vi "Connection Handler.vi"(6 "connection reference":refnum<data-value>, 8 "UUID":string, 9 "Data Model":refnum<class "Device Data Model.lvclass">, 11 "TCP Server":refnum<class "TCP Server.lvclass">) -> ()   [LabVIEW 2021, in "WebSockets.lvlib" / "TCP Server.lvclass"]
doc: "Handles new connections by waiting on TCP requests. When data is received, it will execute the modbus data unit and write the return data back onto the bus. It handles one request at a time."
uses:
  TCP Server.lvclass
  D:/my_projects/projects/21/WebSockets/Source/WebSockets/WebSocket/WebSocket.lvclass
  Connection.ctl
  Modbus_v121c/Data Model/Device Data Model.lvclass
  TCP Server.lvclass/TCP Server.ctl
  WebSocket/WebSocket.lvclass/WebSocket.ctl
  Data Model/WebSocket Data Model.lvclass
  Data Model/WebSocket Data Model.lvclass/WebSocket Data Model.ctl
  WebSocket/Opcodes.ctl
  Handler State.ctl
  WebSocket/Low-Level Write.vi
  WebSocket/Low-Level Read.vi
  Timing/Calculate Timeout.vi
  WebSocket/Pong.vi
  Timing/Tick Count with Error Wires.vi
  WebSocket/DataLengthBytes.vi
  WebSocket/EncodeMaskedBytes.vi
  WebSocket/Socket Write.vi
  WebSocket/Socket Read.vi
  <vilib>/Utility/error.llb/Error Cluster From Error Code.vi
  WebSocket/DecodeMaskedBytes.vi
  WebSocket/WebSocket.lvclass
  Sockets/Socket/Socket.lvclass
panel:
  out "error out":errorcluster
  out "Data":u8[](array[numeric])
  in  "stop":bool
  # "ToDo: Delete indicator"
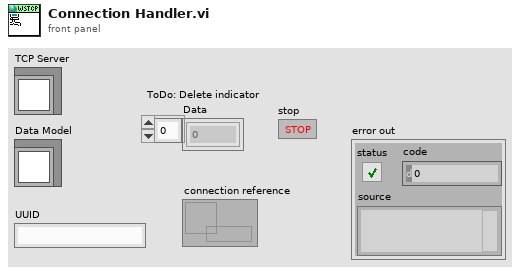
[diagram p1: front panel]
types:
  T1 = typedef "WebSockets.lvlib/WebSocket.lvclass/Opcodes.ctl" = u8
  T2 = typedef "WebSockets.lvlib/TCP Server.lvclass/Handler State.ctl" = enum16{"Wait on Connection", "Execute function", "Close Connection", "Quit"}
  T3 = typedef "WebSockets.lvlib/TCP Server.lvclass/Connection.ctl" = cluster{"Connected?":bool, "IP address":string, "connection error":errorcluster}
  T4 = typedef "WebSockets.lvlib/TCP Server.lvclass/Connection Counter.ctl" = cluster{"Currently Connected":u32, "Connection Records":refnum<data-value>[]}
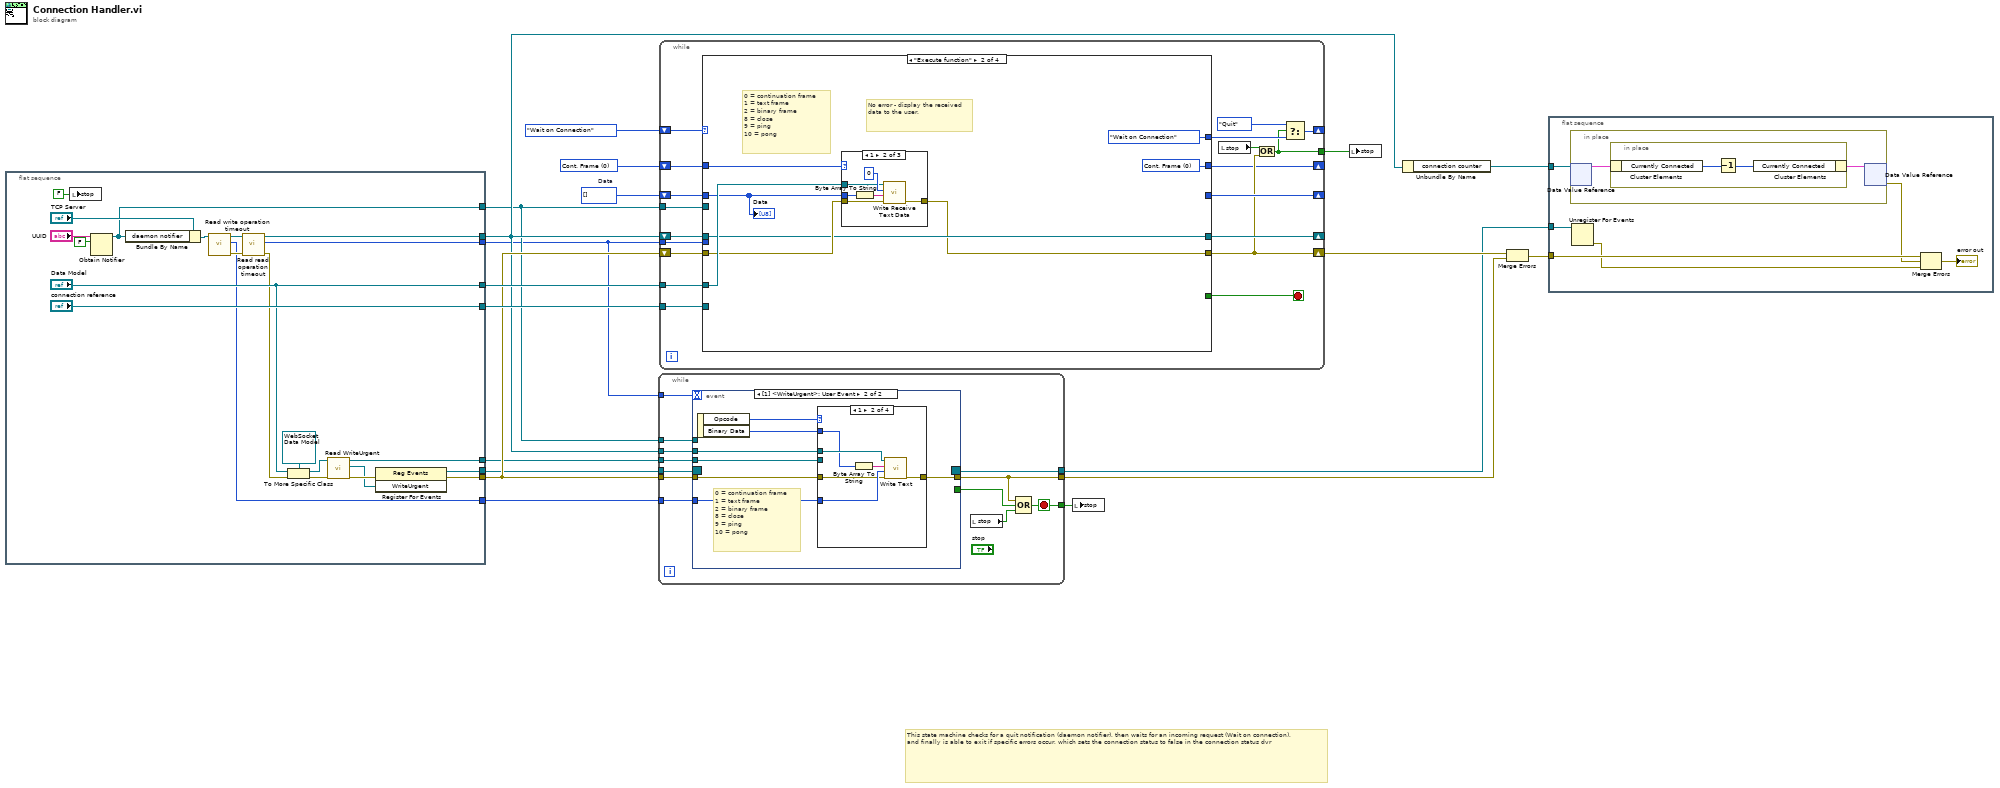
[diagram p0: block diagram]
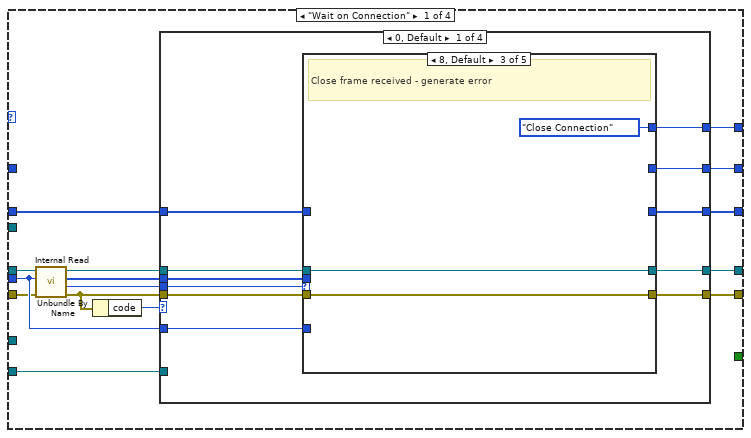
[diagram p2: hidden frame]
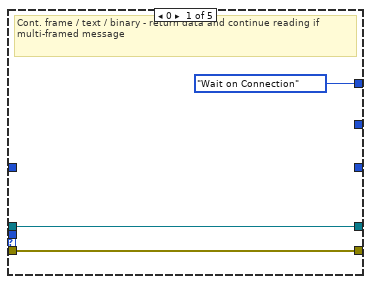
[diagram p3: hidden frame]
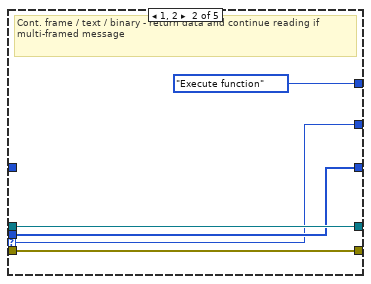
[diagram p4: hidden frame]
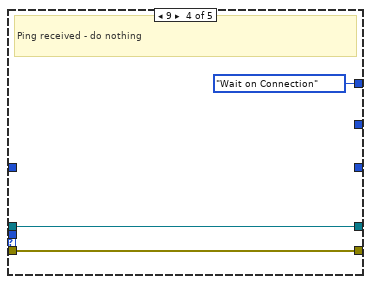
[diagram p5: hidden frame]
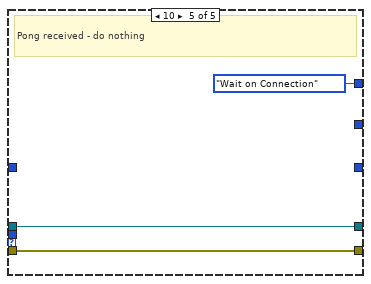
[diagram p6: hidden frame]
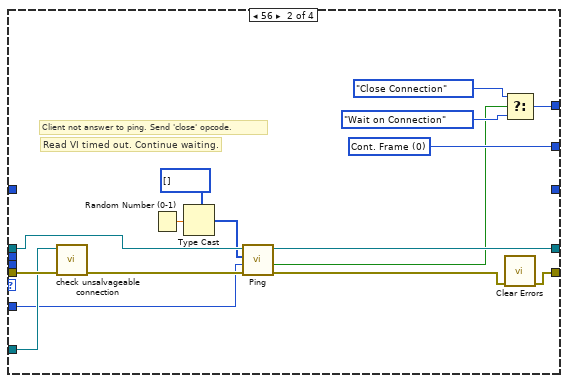
[diagram p7: hidden frame]
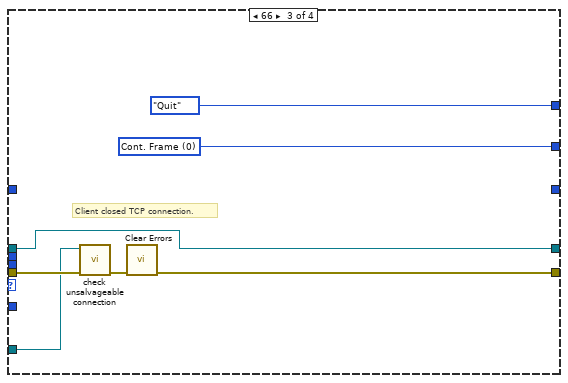
[diagram p8: hidden frame]
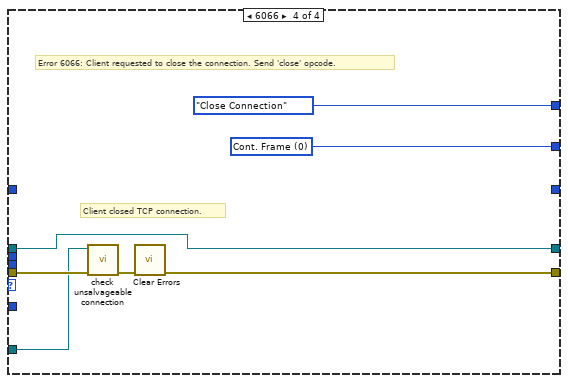
[diagram p9: hidden frame]
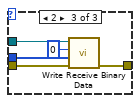
[diagram p11: hidden frame]
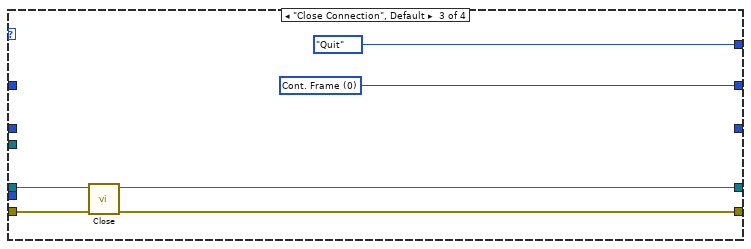
[diagram p12: hidden frame]
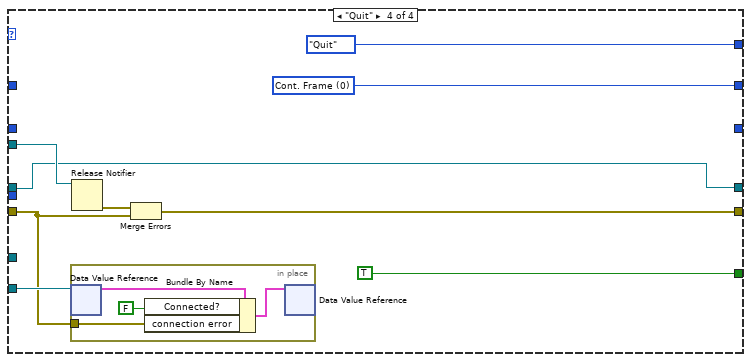
[diagram p13: hidden frame]
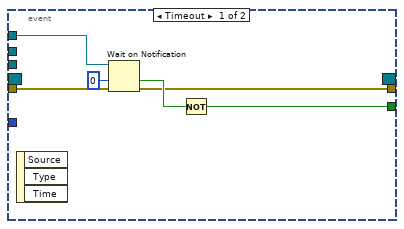
[diagram p14: hidden frame]
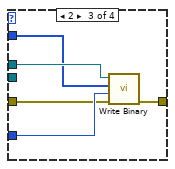
[diagram p16: hidden frame]
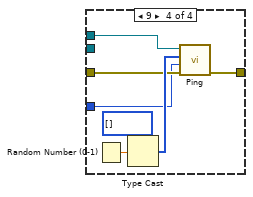
[diagram p17: hidden frame]
diagram:
  w5 = T1 0 items=["Cont. Frame"=0, "Text"=1, "Binary"=2, "Close Frame"=8, "Ping"=9, "Pong"=10] ("Opcode")
  w18 = u8[] []  # Data
  # "This state machine checks for a quit notification (daemon notifier), then waits for an incoming request (Wait on connection), and finally is able to exit if specific errors occur, which sets the connection status to false in the connection status dvr"
  n1 = flat-sequence {
    tunnel: ["connection reference"] -> w16
    tunnel: [w21] -> w12
    tunnel: [w36] -> w3
    tunnel: [w29] -> w11
    tunnel: [w35] -> w4
    tunnel: ["Data Model"] -> w13
    tunnel: [w20] -> w6
    tunnel: [w26] -> w9
    tunnel: [w24] -> w10
    frame #0 {
      n2 = local write "stop"(FALSE ("stop")) -> ()
      n3 = Obtain Notifier(name (unnamed)="UUID", notification data type=FALSE) -> (notifier out=w35:refnum<notifier>)  [unwired: 2 in, 2 out]
      n4 = Bundle By Name(cluster="TCP Server", "daemon notifier"=w35) -> (w30:refnum<class "TCP Server.lvclass">)
      n5 = call "Read write operation timeout.vi"("Socket in"=w30) -> ("error out"=w27:errorcluster, "write operation timeout"=w26:i32, "Socket out"=w28:refnum<class "TCP Server.lvclass">)  [unwired: 8 in]
      n6 = call "Read read operation timeout.vi"("error in (no error)"=w27, "Socket in"=w28) -> ("error out"=w25:errorcluster, "read operation timeout"=w36:i32, "Socket out"=w29:refnum<class "TCP Server.lvclass">)  [unwired: 7 in]
      n7 = To More Specific Class(target class=refnum<class "WebSocket Data Model.lvclass"> refnum ("WebSockets.lvlib:Device Data Model"), reference="Data Model", error in=w25) -> (specific class reference=w32:refnum<class "WebSocket Data Model.lvclass">, error out=w31:errorcluster)
      n8 = call "Read WriteUrgent.vi"("error in (no error)"=w31, "WebSocket Data Model in"=w32) -> ("error out"=w23:errorcluster, "WriteUrgent"=w22:refnum<user-event>, "WebSocket Data Model out"=w24:refnum<class "WebSocket Data Model.lvclass">)  [unwired: 7 in]
      n9 = register-events(error in=w23, w22) -> (reference out=w20:refnum<event-registration>, error out=w21:errorcluster)  [unwired: 1 in]
    }
  }
  n10 = while {
    tunnel: [w52] -> w8
    tunnel: [w43] -> w7
    tunnel: w6 -> [w47]
    tunnel: w12 -> [w51]
    tunnel: w11 -> [w50]
    tunnel: w10 -> [w49]
    tunnel: w9 -> [w48]
    tunnel: w4 -> [w46]
    tunnel: w3 -> [w45]
    tunnel: [w42] -> w2
    stop <- w52 stop-if-true
    n11 = event shown="[1] <WriteUrgent>: User Event" {
      selector: w47 -> [_ _]
      dyn-events: [_ _] -> w42
      timeout: w45 -> [_ _]
      tunnel: w51 -> [w56 w62]
      tunnel: w50 -> [_ w66]
      tunnel: w49 -> [_ w65]
      tunnel: [w55 w64] -> w43
      tunnel: w48 -> [_ w63]
      tunnel: w46 -> [w59 _]
      tunnel: [w57 _] -> w44
      event Timeout {
        n12 = event-data() -> ()  [unwired: 1 in, 3 out]
        n13 = Wait on Notification(notifier=w59, timeout in ms (-1)=0, error in (no error)=w56) -> (timed out?=w58:bool, error out=w55:errorcluster)  [unwired: 1 in, 2 out]
        n14 = Not(x=w58) -> (.not. x?=w57:bool)
      }
      event User Event {
        # "0 = continuation frame\n1 = text frame\n2 = binary frame\n8 = close\n9 = ping\n10 = pong"
        n15 = event-data() -> ("Opcode"=w61:T1, "Binary Data"=w60:u8[])  [unwired: 1 in]
        n16 = case shown="1" w61 {
          tunnel: w66 -> [_ w73 w78 w83]
          tunnel: w62 -> [w67 w69 w74 w81]
          tunnel: w65 -> [_ _ _ _]
          tunnel: w63 -> [_ w72 w76 w79]
          tunnel: [w67 w71 w77 w80] -> w64
          tunnel: w60 -> [_ w70 w75 _]
          frame 0, Default {
          }
          frame 1 {
            n17 = Byte Array To String(unsigned byte array=w70) -> (string=w68:string)
            n18 = call-dynamic "Write Text.vi"("error in (no error)"=w69, "timeout ms (5000)"=w72, "String Data"=w68, "WebSocket in"=w73) -> ("error out"=w71:errorcluster)  [unwired: 6 in, 1 out]
          }
          frame 2 {
            n19 = call-dynamic "Write Binary.vi"("error in (no error)"=w74, "timeout ms (5000)"=w76, "Binary Data"=w75, "WebSocket in"=w78) -> ("error out"=w77:errorcluster)  [unwired: 6 in, 1 out]
          }
          frame 9 {
            n20 = Random Number (0-1)() -> (number: 0 to 1=w84:dbl)
            n21 = Type Cast(type=u8[] [] ("values"), x=w84) -> (*(type *) &x=w82:u8[])
            n22 = call "Ping.vi"("error in (no error)"=w81, "timeout ms (5000)"=w79, "Payload"=w82, "WebSocket in"=w83) -> ("error out"=w80:errorcluster)  [unwired: 5 in, 2 out]
          }
        }
      }
    }
    n23 = local read "stop"() -> (w53:bool)
    n24 = Compound Arithmetic op=OR(w43, w44, w53) -> (w52:bool)
  }
  n25 = while {
    tunnel: w3 -> [w102]
    shift-right: [w103] -> _
    shift-left: w11 -> [w104]
    shift-right: [w100] -> _
    shift-left: w18 -> [w101]
    shift-right: [w91] -> _
    shift-left: Handler_State."Wait on Connection" ("Listener State") -> [w98]
    tunnel: w16 -> [w99]
    tunnel: w4 -> [w96]
    tunnel: [w89] -> w15
    shift-right: [w90] -> w14
    shift-left: w12 -> [w97]
    tunnel: w13 -> [w88]
    shift-right: [w87] -> _
    shift-left: w5 -> [w86]
    stop <- w95 stop-if-true
    n26 = case shown="\"Execute function\"" w98 {
      tunnel: w104 -> [w112 w181 w202 w207]
      tunnel: [w119 w180 w199 w211] -> w90
      tunnel: [w118 w181 w200 w207] -> w103
      tunnel: [_ _ _ TRUE ("Finished?")] -> w95
      tunnel: w102 -> [w109 _ _ _]
      tunnel: w101 -> [w117 w183 _ _]
      tunnel: [w116 _ _ _] -> w100
      tunnel: w99 -> [w114 _ _ w209]
      tunnel: [w113 Handler_State."Wait on Connection" ("Listener State") Handler_State."Quit" ("Listener State") Handler_State."Quit" ("Listener State")] -> w92
      tunnel: w97 -> [w108 w182 w203 w205]
      tunnel: w96 -> [_ _ _ w210]
      tunnel: w88 -> [_ w184 _ _]
      tunnel: [w105 w179 w198 w204] -> w87
      tunnel: w86 -> [_ w178 _ _]
      frame "Wait on Connection" {
        n27 = call "Internal Read.vi"("error in (no error)"=w108, "timeout ms"=w109, "WebSocket in"=w112) -> ("error out"=w107:errorcluster, "Opcode"=w106:T1, "Data"=w110:u8[], "WebSocket out"=w111:refnum<class "TCP Server.lvclass">)  [unwired: 5 in]
        n28 = Unbundle By Name(w107) -> ("code"=w115:i32)
        n29 = case shown="0, Default" w115 {
          tunnel: w107 -> [w130 w163 w169 w176]
          tunnel: [w129 w161 w167 w174] -> w119
          tunnel: w111 -> [w128 w160 w166 w173]
          tunnel: w110 -> [w127 _ _ _]
          tunnel: [w126 w149 w166 w173] -> w118
          tunnel: w106 -> [w125 _ _ _]
          tunnel: w109 -> [w124 w158 _ _]
          tunnel: w117 -> [w123 _ _ _]
          tunnel: [w122 _ _ _] -> w116
          tunnel: w114 -> [_ w162 w168 w175]
          tunnel: [w121 w155 Handler_State."Quit" ("Listener State") Handler_State."Close Connection" ("Listener State")] -> w113
          tunnel: [w120 w154 w164 w171] -> w105
          frame 0, Default {
            n30 = case shown="8, Default" w125 {
              selector: w125 -> [_ w134 _ _ _]
              tunnel: w130 -> [w132 w137 w141 w142 w146]
              tunnel: [w132 w137 w141 w142 w146] -> w129
              tunnel: w128 -> [w133 w138 w140 w143 w147]
              tunnel: w127 -> [_ w136 _ _ _]
              tunnel: [w133 w138 w140 w143 w147] -> w126
              tunnel: w124 -> [_ _ _ _ _]
              tunnel: w123 -> [_ _ _ _ _]
              tunnel: [_ w136 _ _ _] -> w122
              tunnel: [Handler_State."Wait on Connection" ("Listener State") Handler_State."Execute function" ("Listener State") Handler_State."Close Connection" ("Listener State") Handler_State."Wait on Connection" ("Listener State") Handler_State."Wait on Connection" ("Listener State")] -> w121
              tunnel: [_ w134 _ _ _] -> w120
              frame 0 {
                # "Cont. frame / text / binary - return data and continue reading if multi-framed message"
              }
              frame 1, 2 {
                # "Cont. frame / text / binary - return data and continue reading if multi-framed message"
              }
              frame 8, Default {
                # "Close frame received - generate error"
              }
              frame 9 {
                # "Ping received - do nothing"
              }
              frame 10 {
                # "Pong received - do nothing"
              }
            }
          }
          frame 56 {
            w154 = T1 0 items=["Cont. Frame", "Text", "Binary", "Close Frame", "Ping", "Pong"] ("Opcode")
            # "Client not answer to ping. Send 'close' opcode."
            # "Read VI timed out. Continue waiting."
            n31 = call "check unsalvageable connection.vi"("error in (no error)"=w163, "connection reference"=w162) -> ("error out"=w159:errorcluster)  [unwired: 9 in]
            n32 = Random Number (0-1)() -> (number: 0 to 1=w152:dbl)
            n33 = Type Cast(type=u8[] [] ("values"), x=w152) -> (*(type *) &x=w151:u8[])
            n34 = call "Ping.vi"("error in (no error)"=w159, "timeout ms (5000)"=w158, "Payload"=w151, "WebSocket in"=w160) -> ("error out"=w150:errorcluster, "timed out?"=w148:bool, "WebSocket out"=w149:refnum<class "TCP Server.lvclass">)  [unwired: 5 in]
            n35 = Select(t=Handler_State."Close Connection" ("Listener State"), s=w148, f=Handler_State."Wait on Connection" ("Listener State")) -> (s? t:f=w155:T2)
            n36 = call <vilib>:"Clear Errors.vi"("error in (no error)"=w150) -> ("error out"=w161:errorcluster)  [unwired: 5 in, 1 out]
          }
          frame 66 {
            w164 = T1 0 items=["Cont. Frame", "Text", "Binary", "Close Frame", "Ping", "Pong"] ("Opcode")
            # "Client closed TCP connection."
            n37 = call "check unsalvageable connection.vi"("error in (no error)"=w169, "connection reference"=w168) -> ("error out"=w170:errorcluster)  [unwired: 9 in]
            n38 = call <vilib>:"Clear Errors.vi"("error in (no error)"=w170) -> ("error out"=w167:errorcluster)  [unwired: 5 in, 1 out]
          }
          frame 6066 {
            w171 = T1 0 items=["Cont. Frame", "Text", "Binary", "Close Frame", "Ping", "Pong"] ("Opcode")
            # "Error 6066: Client requested to close the connection. Send 'close' opcode."
            # "Client closed TCP connection."
            n39 = call "check unsalvageable connection.vi"("error in (no error)"=w176, "connection reference"=w175) -> ("error out"=w177:errorcluster)  [unwired: 9 in]
            n40 = call <vilib>:"Clear Errors.vi"("error in (no error)"=w177) -> ("error out"=w174:errorcluster)  [unwired: 5 in, 1 out]
          }
        }
      }
      frame "Execute function" {
        w179 = T1 0 items=["Cont. Frame", "Text", "Binary", "Close Frame", "Ping", "Pong"] ("Opcode")
        # "0 = continuation frame\n1 = text frame\n2 = binary frame\n8 = close\n9 = ping\n10 = pong"
        # "No error - display the received data to the user."
        n41 = case shown="1" w178 {
          tunnel: w183 -> [_ w192 w194]
          tunnel: w184 -> [_ w188 w195]
          tunnel: w182 -> [w186 w191 w197]
          tunnel: [w186 w187 w196] -> w180
          frame 0, Default {
          }
          frame 1 {
            n42 = Byte Array To String(unsigned byte array=w192) -> (string=w189:string)
            n43 = call-dynamic "Write Receive Text Data.vi"("error in (no error)"=w191, "values"=w189, "starting address"=u16 0, "standard data model in"=w188) -> ("error out"=w187:errorcluster)  [unwired: 6 in, 1 out]
          }
          frame 2 {
            n44 = call-dynamic "Write Receive Binary Data.vi"("error in (no error)"=w197, "values"=w194, "starting address"=u16 0, "standard data model in"=w195) -> ("error out"=w196:errorcluster)  [unwired: 6 in, 1 out]
          }
        }
        "Data" <- w183
      }
      frame "Close Connection", Default {
        w198 = T1 0 items=["Cont. Frame", "Text", "Binary", "Close Frame", "Ping", "Pong"] ("Opcode")
        n45 = call-dynamic "Close.vi"("error in (no error)"=w203, "WebSocket in"=w202) -> ("error out"=w199:errorcluster, "WebSocket out"=w200:refnum<class "TCP Server.lvclass">)  [unwired: 8 in]
      }
      frame "Quit" {
        w204 = T1 0 items=["Cont. Frame", "Text", "Binary", "Close Frame", "Ping", "Pong"] ("Opcode")
        n46 = in-place {
          in-place-border: w205 -> [w213]
          n47 = in-place-dvr #1(w209) -> (w216:T3)  [unwired: 1 out]
          n48 = Bundle By Name(cluster=w216, "Connected?"=FALSE, "connection error"=w213) -> (w214:T3)
          n49 = in-place-dvr #1(w214) -> ()  [unwired: 2 out]
        }
        n50 = Release Notifier(notifier=w210) -> (error out=w206:errorcluster)  [unwired: 2 in, 2 out]
        n51 = Merge Errors(w206, w205) -> (w211:errorcluster)
      }
    }
    n52 = local read "stop"() -> (w94:bool)
    n53 = Or(x=w94, y=w90) -> (x .or. y?=w89:bool)
    n54 = Select(t=Handler_State."Quit" ("Listener State"), s=w89, f=w92) -> (s? t:f=w91:T2)
  }
  n55 = local write "stop"(w8) -> ()
  n56 = local write "stop"(w15) -> ()
  n57 = Unbundle By Name(w11) -> ("connection counter"=w19:refnum<data-value>)
  n58 = Merge Errors(w14, w7) -> (w1:errorcluster)
  n59 = flat-sequence {
    tunnel: w2 -> [w217]
    tunnel: w19 -> [w222]
    tunnel: w1 -> [w221]
    frame #0 {
      n60 = in-place {
        n61 = in-place-dvr #2(w222) -> (w224:T4)  [unwired: 1 out]
        n62 = in-place {
          n63 = in-place-cluster #3(w224) -> ("Currently Connected"=w226:u32)
          n64 = Decrement(x=w226) -> (x-1=w225:u32)
          n65 = in-place-cluster #3("Currently Connected"=w225) -> (w223:T4)
        }
        n66 = in-place-dvr #2(w223) -> (w220:errorcluster)  [unwired: 1 out]
      }
      n67 = Unregister For Events(event registration refnum=w217) -> (error out=w219:errorcluster)  [unwired: 1 in]
      n68 = Merge Errors(w221, w220, w219) -> (→"error out":errorcluster)
    }
  }
